vi "Setup Formatter.vi"(8 "error in":errorcluster) -> (0 "error out":errorcluster, 3 "JSON Serializer out":refnum<class "JSON Serializer.lvclass">)   [LabVIEW 2014]
uses:
  <vilib>/NI/AQ Character Lineator/JSON Serializer/JSON Serializer.lvclass
  <vilib>/NI/AQ Character Lineator/Formatter/Path Embedding.ctl
  <vilib>/NI/AQ Character Lineator/Serialization Common/Serial Version.ctl
  <vilib>/NI/AQ Character Lineator/Formatter/Formatter.lvclass
  <vilib>/NI/AQ Character Lineator/JSON Serializer/JSON Serializer.lvclass/JSON Serializer.ctl
  <vilib>/NI/AQ Character Lineator/Formatter/Formatter.lvclass/Formatter.ctl
  <vilib>/NI/AQ Character Lineator/Serializer/Serializer.lvclass
  <vilib>/NI/AQ Character Lineator/Serialization Common/Serialization Common.lvlib
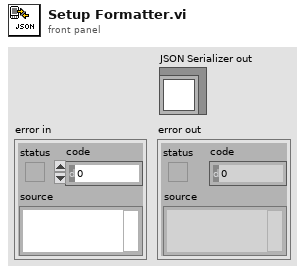
[diagram p1: front panel]
types:
  T1 = typedef "Serialization Common.lvlib/Serial Version.ctl" = cluster{"Major":u16, "Minor":u16, "Fix":u16, "Build":u16}
  T2 = typedef "Formatter.lvclass/Path Embedding.ctl" = enum16{"No paths embedded", "One path with each object", "All paths with each top object"}
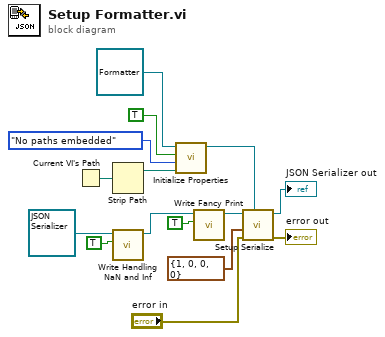
[diagram p0: block diagram]
diagram:
  n1 = Current VI's Path() -> (path=w10:path)
  n2 = Strip Path(path=w10) -> (stripped path=w9:path)  [unwired: 1 out]
  n3 = call <vilib>:"Write Handling NaN and Inf.vi"("Allow encoding NaN and Infinity?"=TRUE, "JSON Serializer in"=refnum<class "JSON Serializer.lvclass"> refnum ("TestSerializer.lvclass")) -> ("JSON Serializer out"=w12:refnum<class "JSON Serializer.lvclass">)  [unwired: 9 in]
  n4 = call <vilib>:"Initialize Properties.vi"("Absolute Path For Dynamic Loading"=w9, "Dynamic Path Behavior"=Path_Embedding."No paths embedded", "Include Default Values? (T)"=TRUE, "Formatter in (Default Formatter)"=refnum<class "Formatter.lvclass"> refnum) -> ("Formatter out"=w14:refnum<class "Formatter.lvclass">)  [unwired: 7 in]
  n5 = call <vilib>:"Write Fancy Print.vi"("Fancy Print"=TRUE, "JSON Serializer in"=w12) -> ("JSON Serializer out"=w11:refnum<class "JSON Serializer.lvclass">)  [unwired: 9 in]
  n6 = call <vilib>:"Setup Serialize.vi"("Formatter (defaults)"=w14, "error in (no error)"="error in", "Serial Version"=T1 {"Major"=1, "Minor"=0, "Fix"=0, "Build"=0}, "Serializer in"=w11) -> ("error out"=→"error out":errorcluster, "Serializer out"=→"JSON Serializer out":refnum<class "JSON Serializer.lvclass">)  [unwired: 6 in]
